vi "Initialize.vi"(8 "error in (no error)":errorcluster, 11 "[V] Tester Parent in":refnum<class "[V] Tester Parent.lvclass">) -> (0 "error out":errorcluster, 3 "[V] Tester Parent out":refnum<class "[V] Tester Parent.lvclass">)   [LabVIEW 2020, in "[V] Tester Parent.lvlib" / "[V] Tester Parent.lvclass"]
uses:
  [V] Tester Parent.lvclass
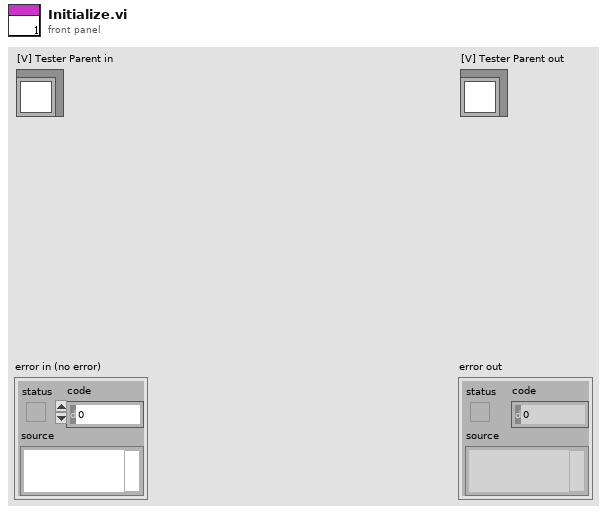
[diagram p1: front panel]
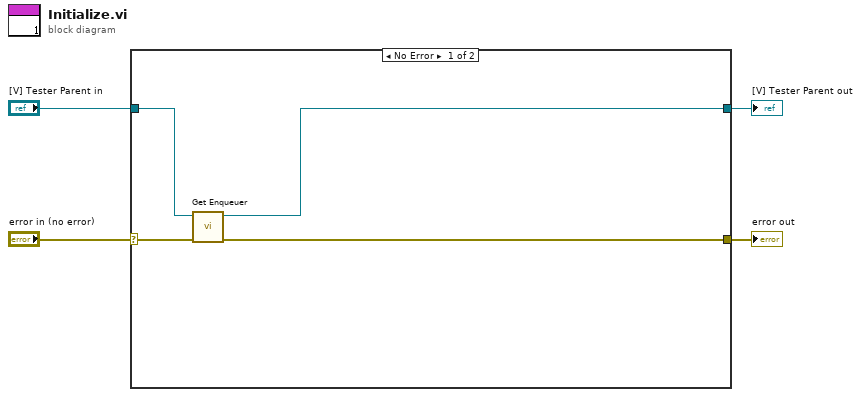
[diagram p0: block diagram]
diagram:
  n1 = case shown="No Error" "error in (no error)" {
    selector: "error in (no error)" -> [w8 w10]
    tunnel: [w7 w10] -> w3
    tunnel: [w5 w9] -> w1
    tunnel: "[V] Tester Parent in" -> [w6 w9]
    frame No Error {
      n2 = call "Get Enqueuer.vi"("error in (no error)"=w8, "[V] Tester Parent in"=w6) -> ("error out"=w7:errorcluster, "[V] Tester Parent out"=w5:refnum<class "[V] Tester Parent.lvclass">)  [unwired: 8 in]
    }
    frame Error {
    }
  }
  "error out" <- w3
  "[V] Tester Parent out" <- w1
